vi "measure_outer.vi"(11 "Qube":refnum<class "System.lvclass">) -> (3 "Qube":refnum<class "System.lvclass">)   [LabVIEW 2021, in "System.lvclass"]
uses:
  System.lvclass
  System.lvclass/System.ctl
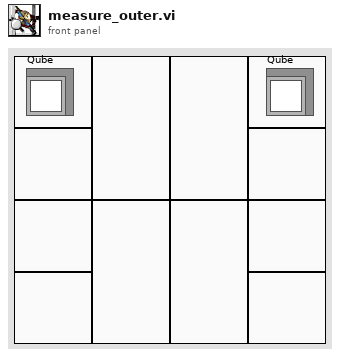
[diagram p1: front panel]
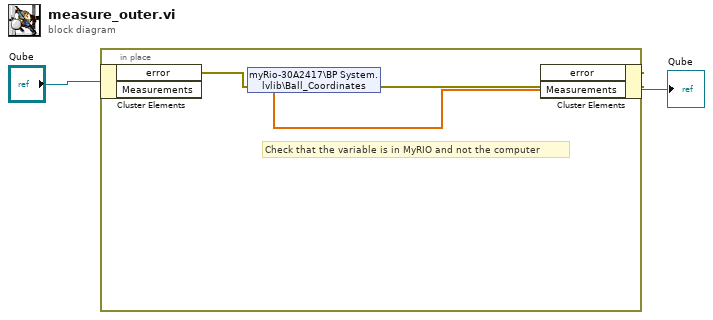
[diagram p0: block diagram]
diagram:
  n1 = in-place {
    # "Check that the variable is in MyRIO and not the computer"
    n2 = in-place-cluster #1("Qube") -> ("error"=w4:errorcluster)  [unwired: 1 out]
    n3 = shared-variable "myRio-30A2417\\BP System.lvlib\\Ball_Coordinates"(error in=w4) -> (w3:dbl[], error out=w5:errorcluster)
    n4 = in-place-cluster #1("error"=w5, "Measurements"=w3) -> (→"Qube":refnum<class "System.lvclass">)
  }
